vi "Close.vi"(8 "error in (no error)":errorcluster caption="错误输入（无错误）", 11 "2601B 输入":refnum<class "2601B.lvclass">) -> (0 "error out":errorcluster caption="错误输出", 3 "2601B 输出":refnum<class "2601B.lvclass">)   [LabVIEW 2020, in "2601B.lvclass"]
uses:
  2601B.lvclass
  2601B.lvclass/2601B.ctl
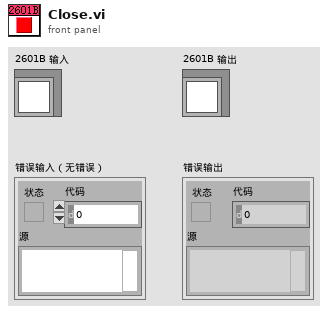
[diagram p1: front panel]
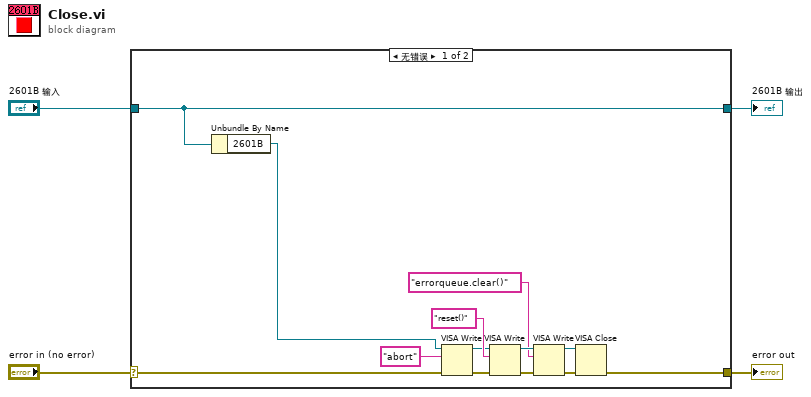
[diagram p0: block diagram]
diagram:
  n1 = case shown="无错误" "error in (no error)" {
    selector: "error in (no error)" -> [w11 w19]
    tunnel: [w17 w19] -> w3
    tunnel: [w16 w18] -> w1
    tunnel: "2601B 输入" -> [w16 w18]
    frame No Error {
      n2 = Unbundle By Name(w16) -> ("2601B"=w9:refnum<visa-resource-name>)
      n3 = VISA Write(VISA resource name=w9, write buffer="abort" ("写入缓冲区"), error in (no error)=w11) -> (VISA resource name out=w14:refnum<visa-resource-name>, error out=w13:errorcluster)  [unwired: 1 out]
      n4 = VISA Write(VISA resource name=w14, write buffer="reset()" ("写入缓冲区"), error in (no error)=w13) -> (VISA resource name out=w7:refnum<visa-resource-name>, error out=w10:errorcluster)  [unwired: 1 out]
      n5 = VISA Write(VISA resource name=w7, write buffer="errorqueue.clear()" ("写入缓冲区"), error in (no error)=w10) -> (VISA resource name out=w6:refnum<visa-resource-name>, error out=w8:errorcluster)  [unwired: 1 out]
      n6 = VISA Close(VISA resource name=w6, error in (no error)=w8) -> (error out=w17:errorcluster)
    }
    frame Error {
    }
  }
  "error out" <- w3
  "2601B 输出" <- w1
